vi "Read XML_Parse RT messageBuffers.vi"(8 "error in (no error)":errorcluster, 11 "remoteTerminal in":refnum<k24>) -> (0 "error out":errorcluster, 2 "RT":T1, 3 "remoteTerminal out":refnum<k24>)   [LabVIEW 2020, in "Ballard 1553 System Explorer.lvlib"]
uses:
  Ballard 1553 System Explorer.lvlib
  Ballard_RT.ctl
  Ballard_RT subAddress.ctl
  Ballard_RT direction.ctl
  Ballard_RT rtMode.ctl
  Ballard_RT modeCode.ctl
  C:/Users/Administrator/Desktop/GIT/Ballard-MIL-STD-1553-Custom-Device/Source/System Explorer/SubVIs/Parse XML Ballard/1.2/BTIXML_SerDes.dll
  1.2/BTIXML_SerDes.dll
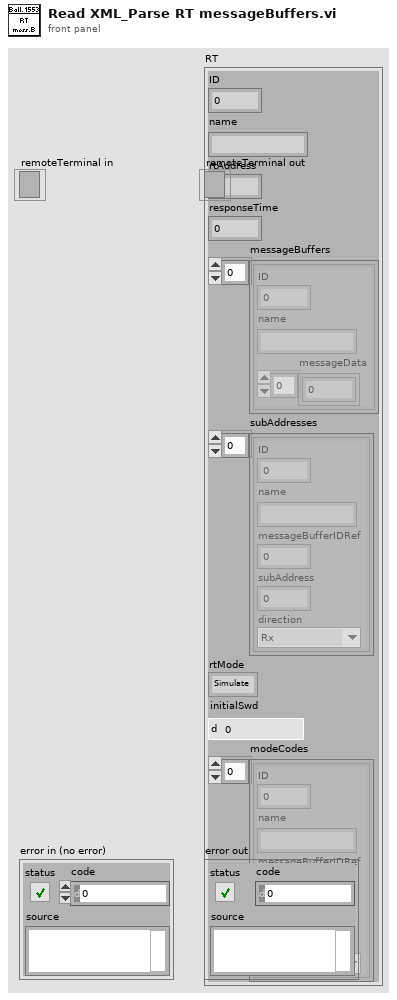
[diagram p1: front panel]
types:
  T1 = typedef "Ballard 1553 System Explorer.lvlib/Ballard_RT.ctl" = cluster{"ID":i32, "name":string, "rtAddress":i8, "responseTime":i32, "messageBuffers":cluster{"ID":i32, "name":string, "messageData":u16[]}[], "subAddresses":T2[], "rtMode":T4, "initialSwd":u16, "modeCodes":T5[]}
  T2 = typedef "Ballard 1553 System Explorer.lvlib/Ballard_RT subAddress.ctl" = cluster{"ID":i32, "name":string, "messageBufferIDRef":i32, "subAddress":i8, "direction":T3}
  T3 = typedef "Ballard 1553 System Explorer.lvlib/Ballard_RT direction.ctl" = enum16{"Tx", "Rx"}
  T4 = typedef "Ballard 1553 System Explorer.lvlib/Ballard_RT rtMode.ctl" = enum16{"Simulate", "Monitor", "Disable"}
  T5 = typedef "Ballard 1553 System Explorer.lvlib/Ballard_RT modeCode.ctl" = cluster{"ID":i32, "name":string, "messageBufferIDRef":i32, "modeCodeNumber":i8, "direction":T3}
  T6 = cluster{"ID":i32, "name":string, "messageData":u16[]}
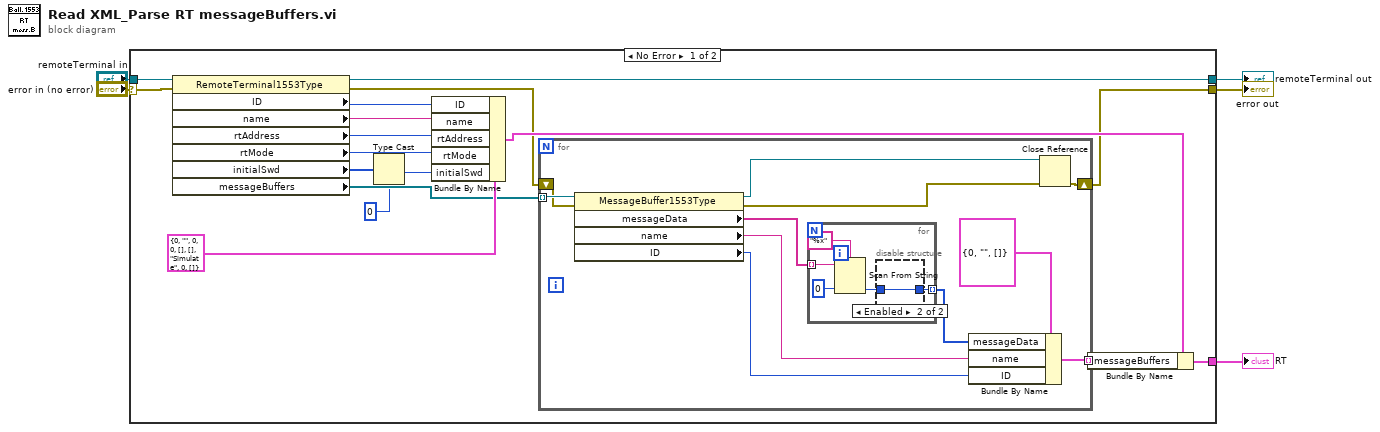
[diagram p0: block diagram]
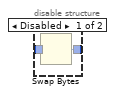
[diagram p2: hidden frame]
diagram:
  n1 = case shown="No Error" "error in (no error)" {
    selector: "error in (no error)" -> [w12 w42]
    tunnel: [w22 _] -> w5
    tunnel: [w6 w42] -> w4
    tunnel: [w21 w43] -> w3
    tunnel: "remoteTerminal in" -> [w14 w43]
    frame No Error {
      n2 = property class="RemoteTerminal1553Type"(reference=w14, error in=w12) -> (reference out=w21:refnum<k24>, error out=w7:errorcluster, "ID"=w17:i32, "name"=w16:string, "rtAddress"=w18:i8, "rtMode"=w13:i32, "initialSwd"=w10:u8[], "messageBuffers"=w11:refnum<k24>[])
      n3 = Type Cast(type=u16 0, x=w10) -> (*(type *) &x=w8:u16)
      n4 = Bundle By Name(cluster=T1 {"ID"=0, "name"="", "rtAddress"=0, "responseTime"=0, "messageBuffers"=[], "subAddresses"=[], "rtMode"=enum."Simulate", "initialSwd"=0, "modeCodes"=[]} ("RT"), "ID"=w17, "name"=w16, "rtAddress"=w18, "rtMode"=w13, "initialSwd"=w8) -> (w19:T1)
      n5 = for {
        tunnel: w11 -> [w33] mode=indexing
        shift-right: [w30] -> w6
        shift-left: w7 -> [w32]
        tunnel: [w23] -> w20 mode=indexing
        n6 = property class="MessageBuffer1553Type"(reference=w33, error in=w32) -> (reference out=w31:refnum<k24>, error out=w29:errorcluster, "messageData"=w28:string[], "name"=w25:string, "ID"=w24:i32)
        n7 = for {
          tunnel: w28 -> [w38] mode=indexing
          tunnel: [w34] -> w26 mode=indexing
          n8 = Scan From String(format string="%x", input string=w38, default 1=u16 0) -> (output 1=w35:u16)  [unwired: 2 in, 3 out]
          n9 = disable-structure shown="Enabled" {
            disable-tunnel: w35 -> [w40 w41]
            disable-tunnel: [w39 w41] -> w34
            frame Disabled {
              n10 = Swap Bytes(anything=w40) -> (byte swapped=w39:u16)
            }
            frame Enabled {
            }
          }
        }
        n11 = Bundle By Name(cluster=T6 {"ID"=0, "name"="", "messageData"=[]} ("messageBuffer"), "messageData"=w26, "name"=w25, "ID"=w24) -> (w23:T6)
        n12 = Close Reference(reference=w31, error in (no error)=w29) -> (error out=w30:errorcluster)
      }
      n13 = Bundle By Name(cluster=w19, "messageBuffers"=w20) -> (w22:T1)
    }
    frame Error {
    }
  }
  "RT" <- w5
  "error out" <- w4
  "remoteTerminal out" <- w3
